vi "读写注册表.vi"(6 "写入内容":string, 7 "键名称":string, 8 "error in (no error)":errorcluster caption="错误输入（无错误）", 11 "读/写":enum16{"读", "写"}(ring)) -> (0 "error out":errorcluster caption="错误输出", 5 "键内容":string caption="字符串/二进制数据")   [LabVIEW 2014]
uses:
  <vilib>/registry/registry.llb/Registry RtKey.ctl
  <vilib>/registry/registry.llb/Read Registry Value Simple STR.vi
  <vilib>/registry/registry.llb/Write Registry Value Simple STR.vi
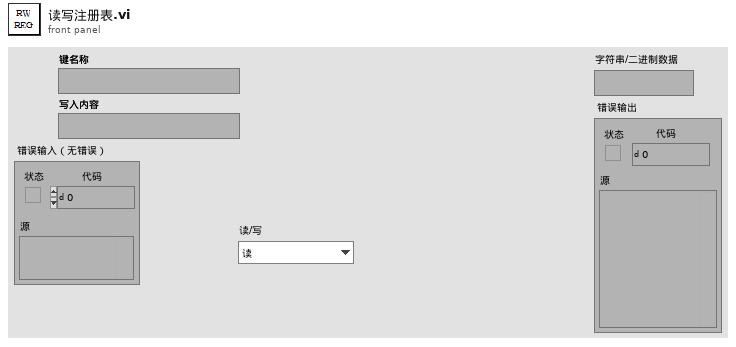
[diagram p1: front panel]
types:
  T1 = typedef "Registry RtKey.ctl" = enum32{"HKEY_CLASSES_ROOT", "HKEY_CURRENT_USER", "HKEY_LOCAL_MACHINE", "HKEY_USERS", "HKEY_PERFORMANCE_DATA", "HKEY_CURRENT_CONFIG", "HKEY_DYN_DATA"}
  T2 = typedef "Registry refnum.ctl" = refnum<k1>
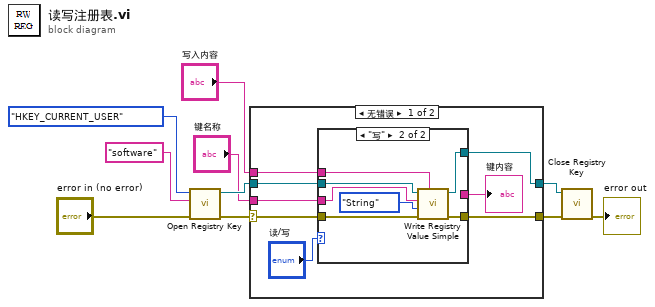
[diagram p0: block diagram]
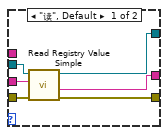
[diagram p2: hidden frame]
diagram:
  n1 = call <vilib>:"Open Registry Key.vi"("error in (no error)"="error in (no error)", "subkey"="software", "root key (HKEY_LOCAL_MACHINE)"=Registry_RtKey."HKEY_CURRENT_USER") -> ("error out"=w8:errorcluster, "refnum out"=w7:T2)  [unwired: 7 in]
  n2 = case shown="无错误" w8 {
    selector: w8 -> [w13 w32]
    tunnel: w7 -> [w17 w33]
    tunnel: "键名称" -> [w16 _]
    tunnel: [w14 w33] -> w3
    tunnel: [w12 w32] -> w4
    tunnel: "写入内容" -> [w11 _]
    frame No Error {
      n3 = case shown="\"写\"" "读/写" {
        tunnel: w17 -> [w24 w31]
        tunnel: w16 -> [w23 w26]
        tunnel: [w22 _] -> w15
        tunnel: [w21 w28] -> w14
        tunnel: w13 -> [w20 w30]
        tunnel: [w19 w29] -> w12
        tunnel: w11 -> [_ w25]
        frame "读", Default {
          n4 = call-poly <vilib>:"Read Registry Value Simple.vi"("error in (no error)"=w20, "value"=w23, "refnum"=w24) -> ("error out"=w19:errorcluster, "String/Binary data"=w22:string, "refnum out"=w21:T2)  [unwired: 3 in, 1 out]
        }
        frame "写" {
          n5 = call-poly <vilib>:"Write Registry Value Simple.vi"("String/Binary data"=w25, "error in (no error)"=w30, "simple data type"=enum16{"String", "Binary", "DWORD"}."String", "value"=w26, "refnum"=w31) -> ("error out"=w29:errorcluster, "refnum out"=w28:T2)  [unwired: 3 in]
        }
      }
      "键内容" <- w15
    }
    frame Error {
    }
  }
  n6 = call <vilib>:"Close Registry Key.vi"("error in (no error)"=w4, "refnum"=w3) -> ("error out"=→"error out":errorcluster)  [unwired: 5 in]
